vi "Error_CtlNotFound.vi"(8 "error in (no error)":errorcluster, 9 "Control Found?":bool, 10 "CtlName":string, 11 "Control in":refnum<vi>) -> (0 "error out":errorcluster, 3 "Control out":refnum<vi>)   [LabVIEW 2020, in "CtlReferences.lvlib" / "CtlReferences.lvclass"]
uses:
  CtlReferences.lvclass
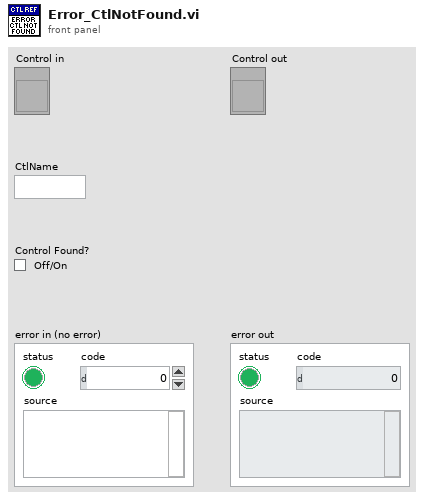
[diagram p1: front panel]
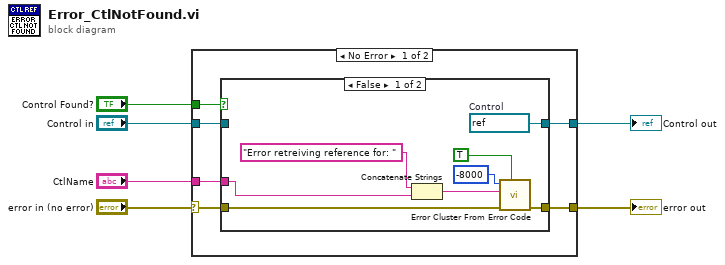
[diagram p0: block diagram]
diagram:
  n1 = case shown="No Error" "error in (no error)" {
    selector: "error in (no error)" -> [w9 w23]
    tunnel: "Control Found?" -> [w12 _]
    tunnel: "CtlName" -> [w11 _]
    tunnel: "Control in" -> [w10 w24]
    tunnel: [w8 w24] -> w2
    tunnel: [w7 w23] -> w1
    frame No Error {
      n2 = case shown="False" w12 {
        tunnel: w9 -> [w14 w22]
        tunnel: [w17 w22] -> w7
        tunnel: [w20 w21] -> w8
        tunnel: w11 -> [w18 _]
        tunnel: w10 -> [_ w21]
        frame False {
          w20 = refnum<vi> refnum  # Control
          n3 = Concatenate Strings("Error retreiving reference for: " ("source"), w18) -> (w16:string)
          n4 = call <vilib>:"Error Cluster From Error Code.vi"("show call chain? (False)"=TRUE ("Force Error? [F]"), "error in (no error)"=w14, "error message (\"\")"=w16, "error code (0)"=-8000 ("code")) -> ("error out"=w17:errorcluster)  [unwired: 5 in]
        }
        frame True {
        }
      }
    }
    frame Error {
    }
  }
  "Control out" <- w2
  "error out" <- w1
